vi "LCA Read Captured Position.vi"(8 "error in (no error)":errorcluster caption="Fehler (Eingang, kein Fehler)", 10 "Position History Index":u8, 11 "Axis Handle":i64) -> (0 "error out":errorcluster caption="Fehler (Ausgang)", 3 "Vaptured Position":dbl)   [LabVIEW 2021, in "labbCAN_MotionControl_API.lvlib"]
doc: "LCA_Func long __stdcall LCA_ReadCapturedPosition(dev_hdl hAxis,\n unsigned char PosHistoryIndex,\n double *pfCapturedPosition);"
uses:
  labbCAN_MotionControl_API.lvlib
  labbCAN_MotionControl_API.dll
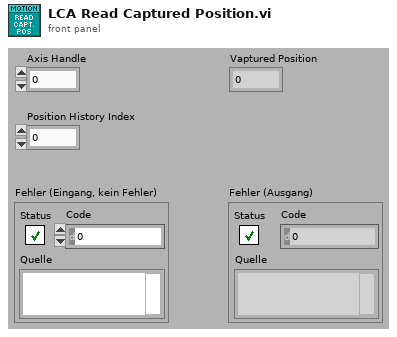
[diagram p1: front panel]
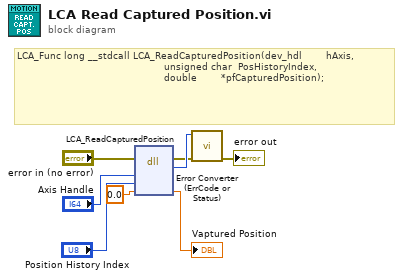
[diagram p0: block diagram]
diagram:
  # "LCA_Func long __stdcall LCA_ReadCapturedPosition(dev_hdl        hAxis,\n                                                 unsigned char  PosHistoryIndex,\n                                                 double        *pfCapturedPosition);"
  n1 = dll-call lib="C:/Users/olaja/AppData/Local/CETONI_SDK/labbCAN_MotionControl_API.*" fn="LCA_ReadCapturedPosition"(error in="error in (no error)", "hAxis"="Axis Handle", "PosHistoryIndex"="Position History Index", "pfCapturedPosition"=0.0) -> (error out=w2:errorcluster, "Rückgabetyp"=w8:i32, "pfCapturedPosition"=→"Vaptured Position":dbl)  [unwired: 4 in, 1 out]
  n2 = call "Error Converter (ErrCode or Status).vi"("error in (no error)"=w2, "error code"=w8) -> ("error out"=→"error out":errorcluster)  [unwired: 9 in]
